vi "Panel.vi"(11 "Team Dashboard Panel in":refnum<class "Team Dashboard Panel.lvclass">) -> ()   [LabVIEW 2020, in "SB App.lvlib" / "Team Dashboard Panel.lvclass"]
uses:
  Team Dashboard Panel.lvclass
  C:/Program Files (x86)/National Instruments/LabVIEW 2020/vi.lib/IlluminatedG/IG OOPanel/OOPanel/Panel/Panel.lvclass
  <vilib>/IlluminatedG/IG OOPanel/OOPanel/Panel/Basic UI State.ctl
  Team Dashboard Panel.lvclass/Team Dashboard Panel.ctl
  SquareBattle/Team/Team.lvclass/Team.ctl
  SquareBattle/Team/Team.lvclass
  <vilib>/IlluminatedG/IG OOPanel/OOPanel/Panel/Panel.lvclass
  <vilib>/IlluminatedG/IG OOPanel/OOPanel/OOPanel.lvlib
  SquareBattle/SquareBattle.lvlib
panel:
  out "Generated":i32
  out "Player Message":string
  out "Collided":i32
  out "Kills":i32
  out "Eliminated":i32
  out "Active":i32
  out "Team Name":string
  out "Color Box":u32(colorbox)
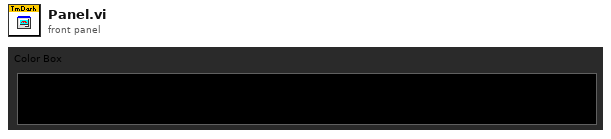
[diagram p1: front panel]
types:
  T1 = typedef "OOPanel.lvlib/Panel.lvclass/Basic UI State.ctl" = enum16{"Init", "Run", "Close"}
  T2 = typedef "SB App.lvlib/Team Dashboard Panel.lvclass/Incoming Events.ctl" = cluster{"Team Status":refnum<user-event>}
  T3 = typedef "OOPanel.lvlib/Panel.lvclass/Panel Events.ctl" = cluster{"Visbility":refnum<user-event>, "Close":refnum<user-event>}
  T4 = typedef "SquareBattle.lvlib/Team State.ctl" = enum16{"Active", "Defeated", "Won"}
  T5 = typedef "SquareBattle.lvlib/Team Stats.ctl" = cluster{"Active":i32, "Generated":i32, "Kills":i32, "Eliminated":i32, "Collided":i32}
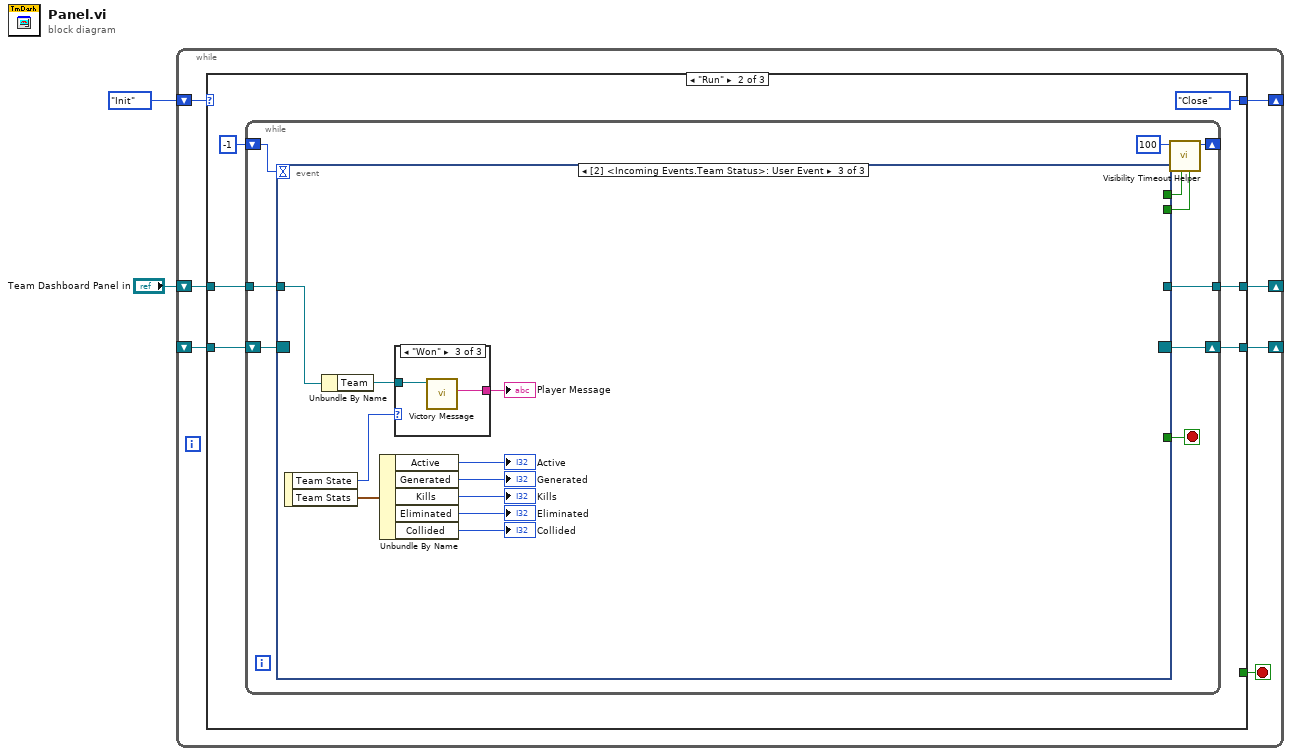
[diagram p0: block diagram]
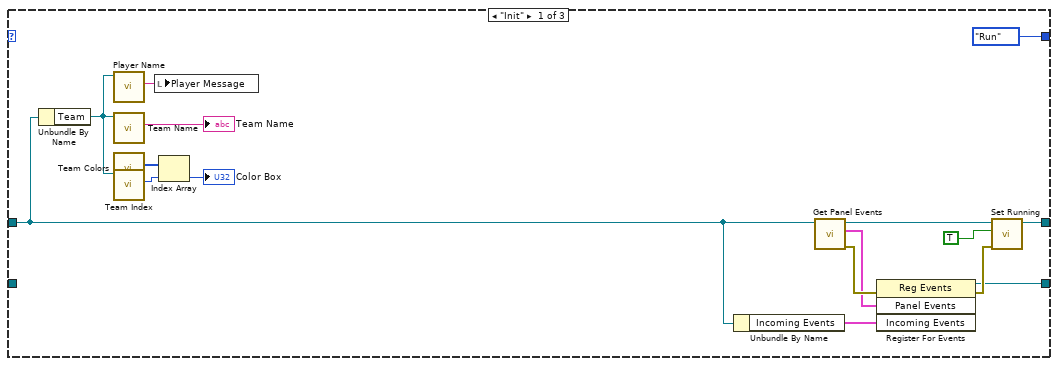
[diagram p2: hidden frame]
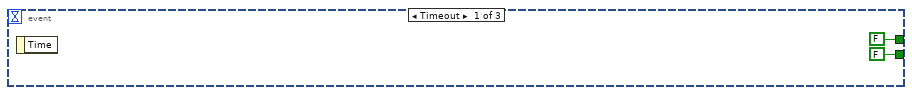
[diagram p3: hidden frame]
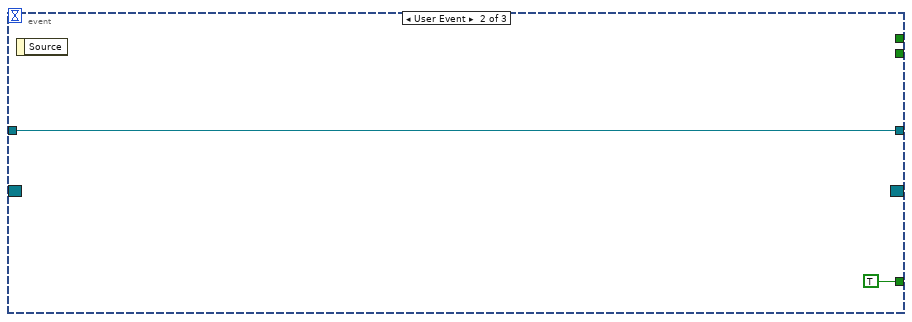
[diagram p4: hidden frame]
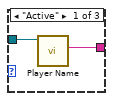
[diagram p5: hidden frame]
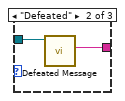
[diagram p6: hidden frame]
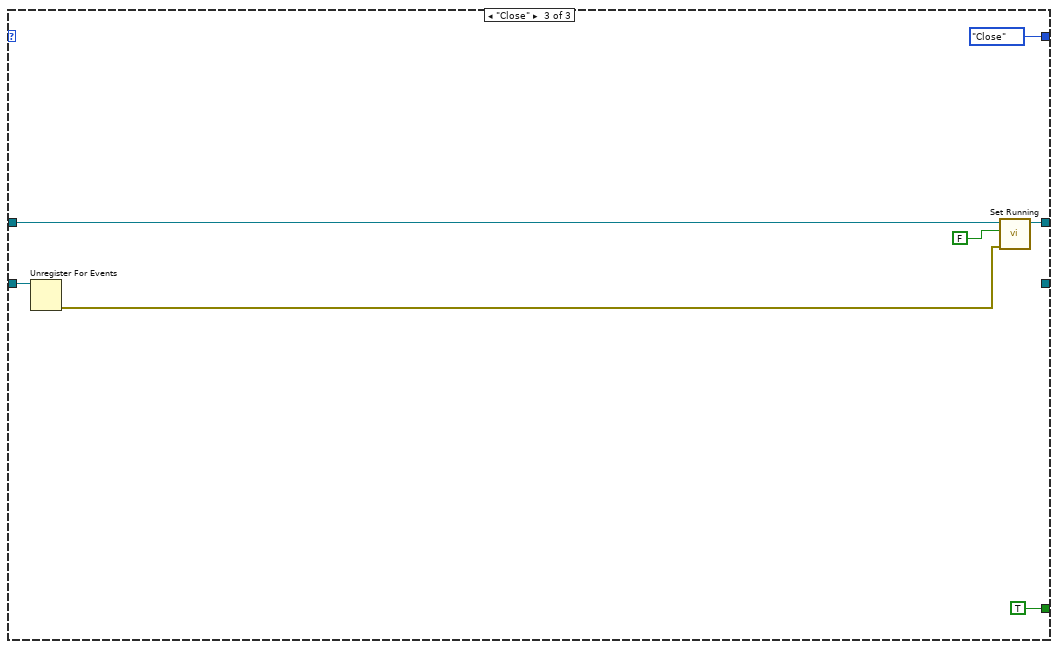
[diagram p7: hidden frame]
diagram:
  n1 = while {
    shift-right: [w8] -> _
    shift-left: _ -> [w9]
    shift-right: [w6] -> _
    shift-left: Basic_UI_State."Init" ("Basic UI State") -> [w7]
    shift-right: [w4] -> _
    shift-left: "Team Dashboard Panel in" -> [w3]
    stop <- w5 stop-if-true
    n2 = case shown="\"Run\"" w7 {
      tunnel: w9 -> [_ w31 w64]
      tunnel: [w19 w29 _] -> w8
      tunnel: [Basic_UI_State."Run" ("Basic UI State") Basic_UI_State."Close" ("Basic UI State") Basic_UI_State."Close" ("Basic UI State")] -> w6
      tunnel: [_ _ TRUE] -> w5
      tunnel: [w18 w26 w62] -> w4
      tunnel: w3 -> [w16 w27 w63]
      frame "Init" {
        n3 = Unbundle By Name(w16) -> ("Team"=w11:refnum<class "Team.lvclass">)
        n4 = call-dynamic "Player Name.vi"("Team"=w11) -> ("Player Name"=w10:string)  [unwired: 10 in]
        n5 = call-dynamic "Team Name.vi"("Team in"=w11) -> ("Team Name"=→"Team Name":string)  [unwired: 10 in]
        n6 = call "Team Colors.vi"() -> ("Team Colors"=w14:u32[])  [unwired: 11 in]
        n7 = call "Team Index.vi"("Team"=w11) -> ("Team Index"=w13:i32)  [unwired: 10 in]
        n8 = local write "Player Message"(w10) -> ()
        n9 = Index Array(array=w14, index=w13) -> (element=→"Color Box":u32)
        n10 = Unbundle By Name(w16) -> ("Incoming Events"=w17:T2)
        n11 = call <vilib>:"Get Panel Events.vi"("Panel in"=w16) -> ("error out"=w25:errorcluster, "Panel Events"=w21:T3, "Panel out"=w22:refnum<class "Team Dashboard Panel.lvclass">)  [unwired: 8 in]
        n12 = register-events(error in=w25, w21, w17) -> (reference out=w19:refnum<event-registration>, error out=w23:errorcluster)  [unwired: 1 in]
        n13 = call <vilib>:"Set Running.vi"("error in (no error)"=w23, "Running"=TRUE, "Panel in"=w22) -> ("Panel out"=w18:refnum<class "Team Dashboard Panel.lvclass">)  [unwired: 7 in, 1 out]
      }
      frame "Run" {
        n14 = while {
          shift-right: [w37] -> w29
          shift-left: w31 -> [w38]
          shift-right: [w40] -> _
          shift-left: -1 ("Timeout") -> [w39]
          tunnel: w27 -> [w33]
          tunnel: [w32] -> w26
          stop <- w34 stop-if-true
          n15 = event shown="[2] <Incoming Events.Team Status>: User Event" {
            selector: w38 -> [_ _ _]
            dyn-events: [_ _ _] -> w37
            timeout: w39 -> [_ _ _]
            tunnel: [FALSE _ _] -> w36
            tunnel: [FALSE _ _] -> w35
            tunnel: [_ TRUE _] -> w34
            tunnel: w33 -> [_ w44 w55]
            tunnel: [_ w44 _] -> w32
            event Timeout {
              n16 = event-data() -> ()  [unwired: 1 in, 1 out]
            }
            event User Event {
              n17 = event-data() -> ()  [unwired: 1 in, 1 out]
            }
            event User Event {
              n18 = event-data() -> ("Team State"=w54:T4, "Team Stats"=w51:T5)  [unwired: 1 in]
              n19 = Unbundle By Name(w55) -> ("Team"=w53:refnum<class "Team.lvclass">)
              n20 = Unbundle By Name(w51) -> ("Active"=→"Active":i32, "Generated"=→"Generated":i32, "Kills"=→"Kills":i32, "Eliminated"=→"Eliminated":i32, "Collided"=→"Collided":i32)
              n21 = case shown="\"Won\"" w54 {
                tunnel: w53 -> [w57 w59 w61]
                tunnel: [w56 w58 w60] -> w52
                frame "Active" {
                  n22 = call-dynamic "Player Name.vi"("Team"=w57) -> ("Player Name"=w56:string)  [unwired: 10 in]
                }
                frame "Defeated" {
                  n23 = call-dynamic "Defeated Message.vi"("Team"=w59) -> ("Defeated Message"=w58:string)  [unwired: 10 in]
                }
                frame "Won" {
                  n24 = call-dynamic "Victory Message.vi"("Team"=w61) -> ("Victory Message"=w60:string)  [unwired: 10 in]
                }
              }
              "Player Message" <- w52
            }
          }
          n25 = call <vilib>:"Visibility Timeout Helper.vi"("Update?"=w35, "Use Timeout?"=w36, "Visible Timeout mS"=100) -> ("Timeout"=w40:i32)  [unwired: 8 in]
        }
      }
      frame "Close" {
        n26 = Unregister For Events(event registration refnum=w64) -> (error out=w66:errorcluster)  [unwired: 1 in]
        n27 = call <vilib>:"Set Running.vi"("error in (no error)"=w66, "Running"=FALSE, "Panel in"=w63) -> ("Panel out"=w62:refnum<class "Team Dashboard Panel.lvclass">)  [unwired: 7 in, 1 out]
      }
    }
  }
